vi "read PID from array.vi"(8 "error in":errorcluster, 10 "loop number":i32, 11 "PID Array":T2) -> (0 "error out":errorcluster, 2 "PID Array Element":T1={"Loop ID"="", "Tags"={"Setpoint"="", "Process Variable"="", "Output"=""}, "Gains"={"P"=1.0, "I"=0.01, "D"=0.0}, "Range"={"High"=100.0, "Low"=-100.0}}, 3 "empty tag?":bool)   [LabVIEW 2013, in "PID Module editor node.lvclass"]
uses:
  PID Module editor node.lvclass
  PID array reference.ctl
  PID array element.ctl
  module/configuration/PID Module configuration.lvclass
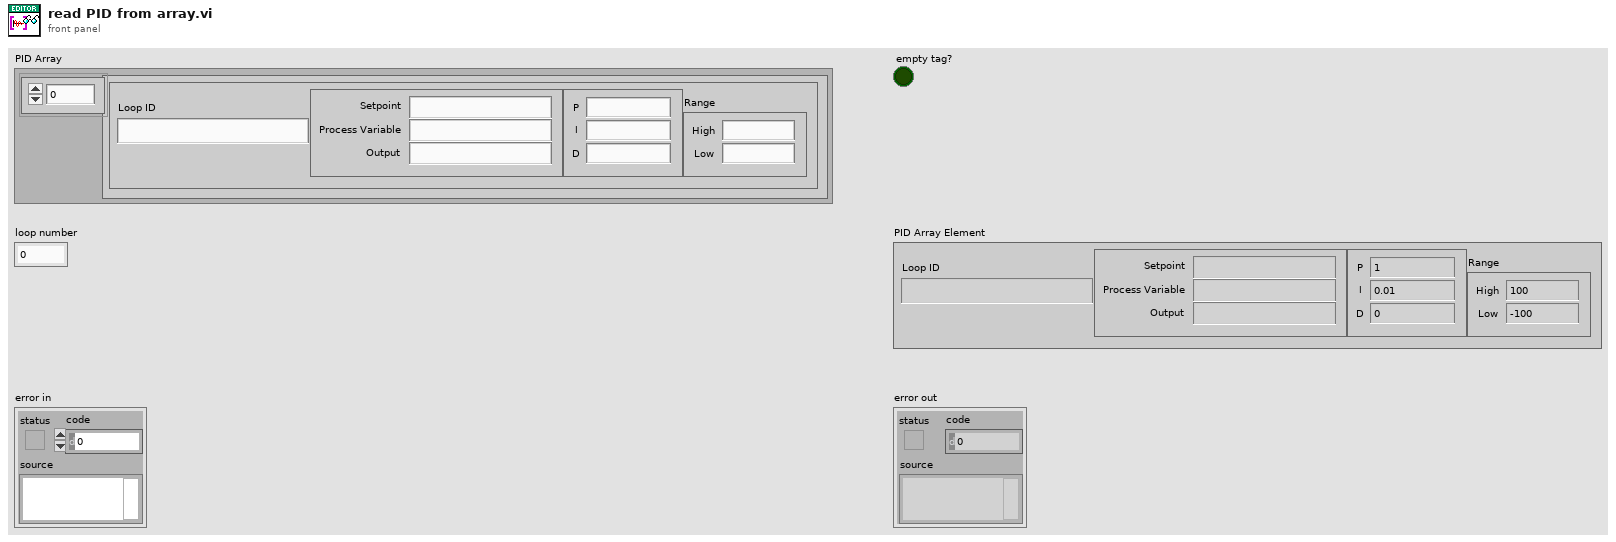
[diagram p1: front panel]
types:
  T1 = typedef "PID Module configuration.lvclass/PID array element.ctl" = cluster{"Loop ID":string, "Tags":cluster{"Setpoint":string, "Process Variable":string, "Output":string}, "Gains":cluster{"P":dbl, "I":dbl, "D":dbl}, "Range":cluster{"High":dbl, "Low":dbl}}
  T2 = typedef "PID Module editor node.lvclass/PID array reference.ctl" = refnum<vi>
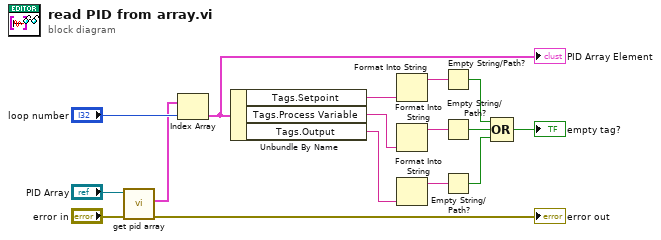
[diagram p0: block diagram]
diagram:
  n1 = call "get pid array.vi"("error in (no error)"="error in", "Array in"="PID Array") -> ("error out"=→"error out":errorcluster, "Value"=w9:T1[])  [unwired: 7 in, 1 out]
  n2 = Index Array(array=w9, index="loop number") -> (element=w8:T1)
  "PID Array Element" <- w8
  n3 = Unbundle By Name(w8) -> ("Tags.Setpoint"=w7:string, "Tags.Process Variable"=w3:string, "Tags.Output"=w4:string)
  n4 = Format Into String(w7) -> (resulting string=w2:string)  [unwired: 3 in, 1 out]
  n5 = Format Into String(w3) -> (resulting string=w6:string)  [unwired: 3 in, 1 out]
  n6 = Format Into String(w4) -> (resulting string=w5:string)  [unwired: 3 in, 1 out]
  n7 = Empty String/Path?(string/path=w2) -> (empty?=w15:bool)
  n8 = Empty String/Path?(string/path=w6) -> (empty?=w14:bool)
  n9 = Empty String/Path?(string/path=w5) -> (empty?=w13:bool)
  n10 = Compound Arithmetic op=OR(w15, w14, w13) -> (→"empty tag?":bool)
